vi "FdxCmdRxTrgLineControlCvi.vi"(8 "error in":errorcluster, 9 "Input Cluster":cluster{"TrgInLine":u32, "TrgOutLine":u32} {"TrgOutLine" items=["FDX_STROBE_LINE_KEEP"=4294967295, "FDX_STROBE_LINE_OFF"=0, "FDX_STROBE_LINE_1"=1, "FDX_STROBE_LINE_2"=2, "FDX_STROBE_LINE_3"=3, "FDX_STROBE_LINE_4"=4]; "TrgInLine" items=["FDX_STROBE_LINE_KEEP"=4294967295, "FDX_STROBE_LINE_OFF"=0, "FDX_STROBE_LINE_1"=1, "FDX_STROBE_LINE_2"=2, "FDX_STROBE_LINE_3"=3, "FDX_STROBE_LINE_4"=4]}, 11 "InstrumentHandle_port":u32) -> (0 "error out":errorcluster, 3 "InstrumentHandle_port":u32)   [LabVIEW 2020, in "AIM664LV.lvlib"]
doc: "This function is used to select the Trigger In- and Output lines for the Receiver part of the associated port."
uses:
  AIM664LV.lvlib
  AFDX_LibraryAdmin/FdxGlobalDllPath.vi
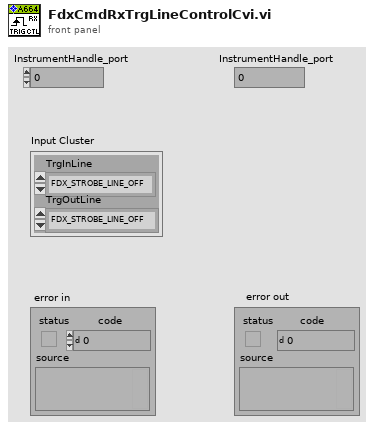
[diagram p1: front panel]
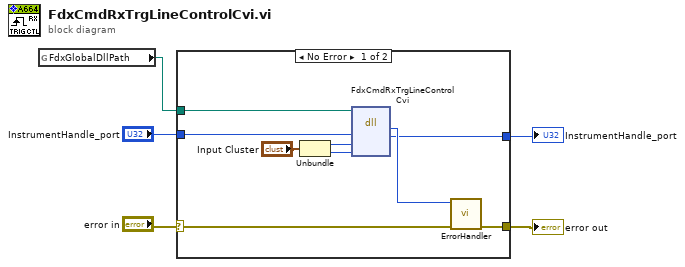
[diagram p0: block diagram]
diagram:
  n1 = global read "FdxGlobalDllPath.vi" "FdxGlobalDllPath"() -> (w3:path)
  n2 = case shown="No Error" "error in" {
    selector: "error in" -> [w13 w16]
    tunnel: [w14 w16] -> w5
    tunnel: w3 -> [w8 _]
    tunnel: "InstrumentHandle_port" -> [w7 w15]
    tunnel: [w6 w15] -> w1
    frame No Error {
      n3 = Unbundle("Input Cluster") -> ("TrgInLine"=w10:u32, "TrgOutLine"=w9:u32)
      n4 = dll-call lib="aim_fdx.19.dll" fn="FdxCmdRxTrgLineControlCvi"(path in=w8, "InstrumentHandle"=w7, "TrgInLine"=w10, "TrgOutLine"=w9) -> ("status"=w12:i32, "InstrumentHandle"=w6:u32)  [unwired: 4 in, 2 out]
      n5 = call "ErrorHandler.vi"("error in"=w13, "AIM Error"=w12) -> ("error out"=w14:errorcluster)  [unwired: 9 in]
    }
    frame Error {
    }
  }
  "error out" <- w5
  "InstrumentHandle_port" <- w1
